vi "data_grid_v128_3d_plot.vi"(9 "No. Rows":i32=16, 10 "No. Columns":i32=8, 11 "Sensor Data":dbl[][](array[numeric])) -> (1 "Y (GRID)":dbl[][](array[numeric]), 2 "X (GRID)":dbl[][](array[numeric]), 3 "Z (GRID)":dbl[][](array[numeric]))   [LabVIEW 2018]
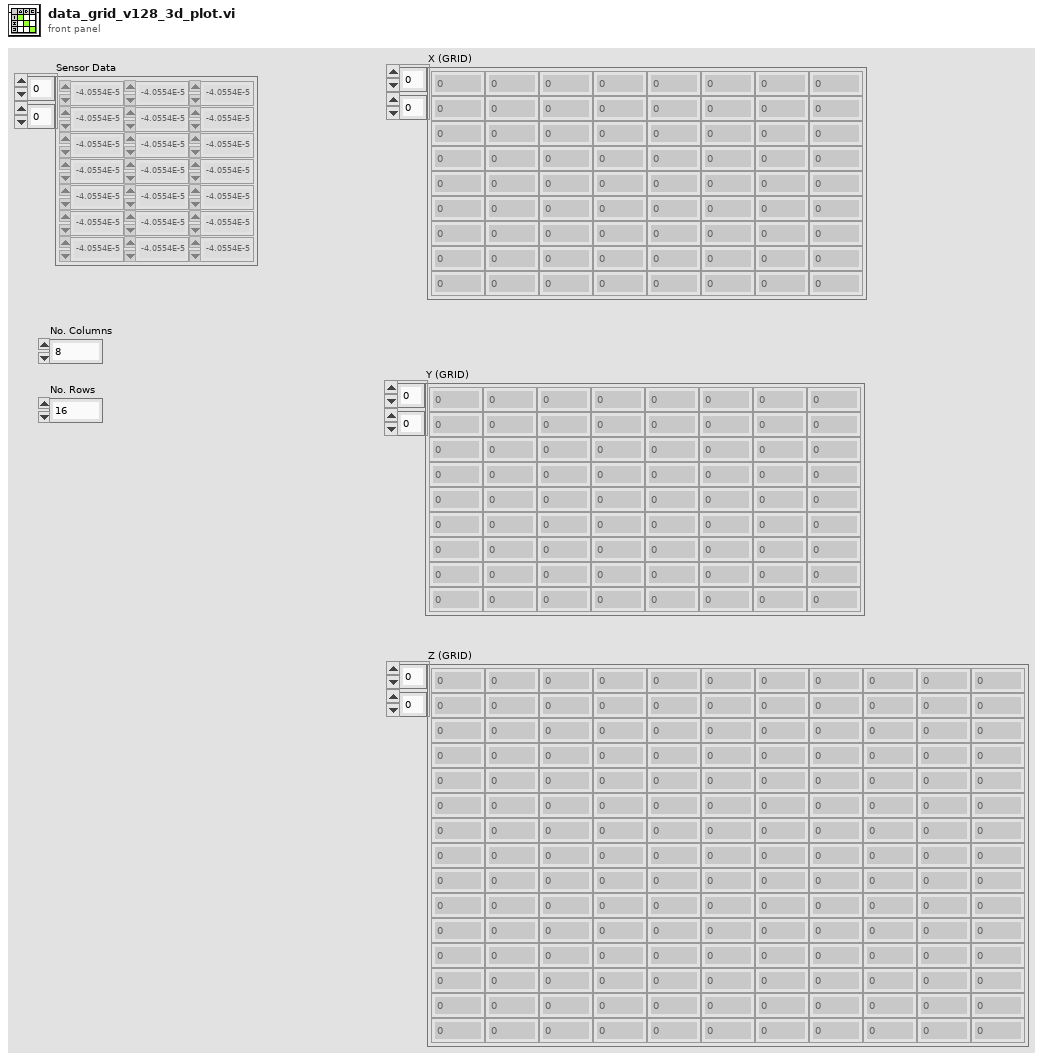
[diagram p1: front panel]
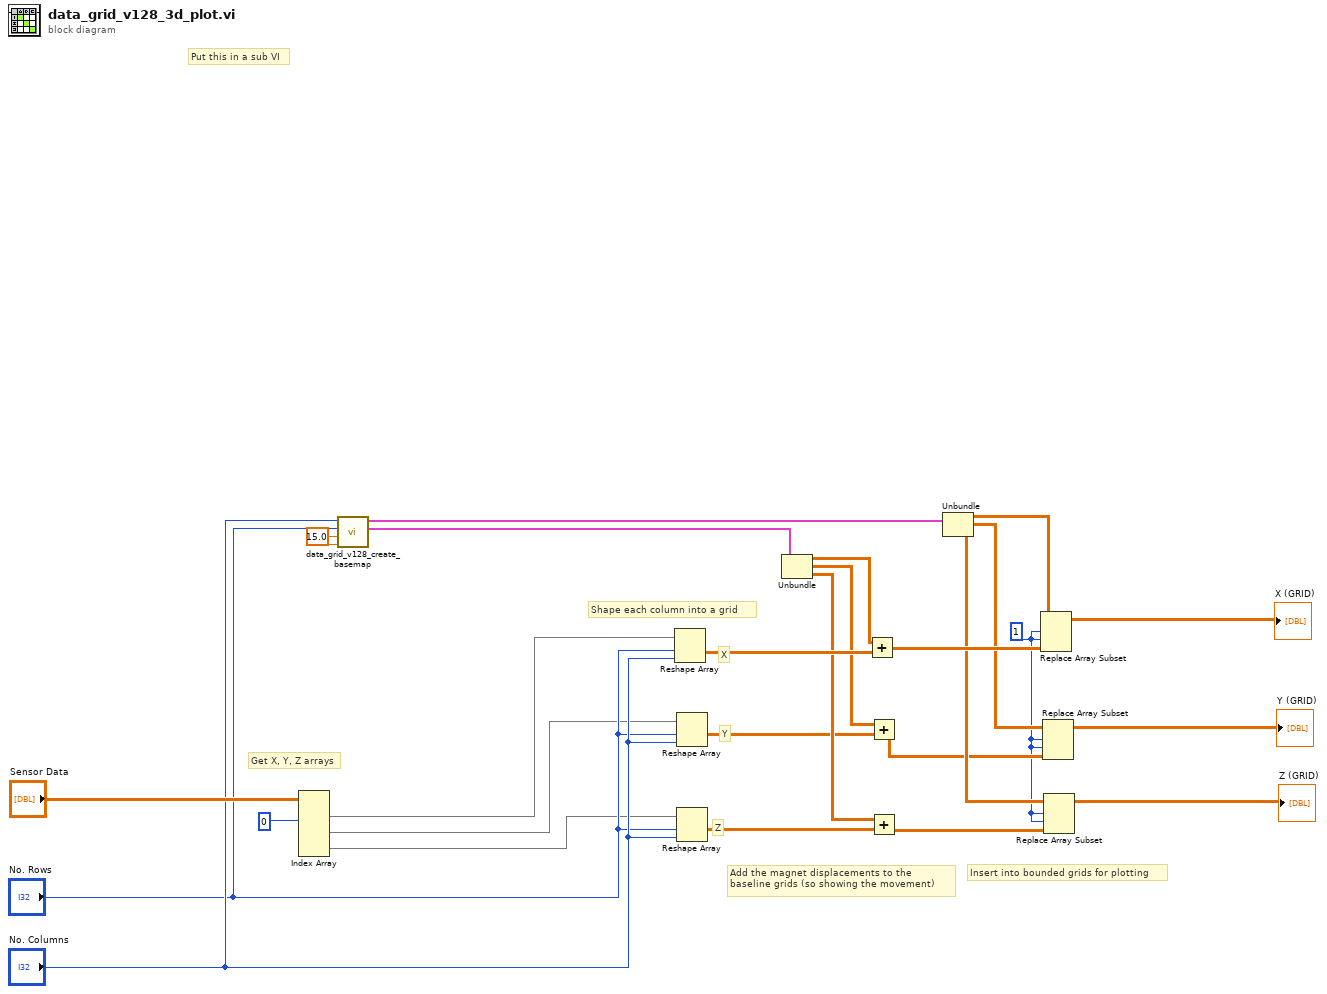
[diagram p0: block diagram]
diagram:
  w6 = 1 ("disabled index (col)")
  w21 = 15.0 ("X_spacing")
  # "Z"
  # "Y"
  # "X"
  # "Insert into bounded grids for plotting"
  # "Add the magnet displacements to the \nbaseline grids (so showing the movement)"
  # "Get X, Y, Z arrays"
  # "Shape each column into a grid"
  # "Put this in a sub VI"
  n1 = Index Array(array="Sensor Data", index (col) #1=0 ("disabled index (col)")) -> (element #1=w24:dbl[], element #2=w2:dbl[], element #3=w1:dbl[])  [unwired: 5 in]
  n2 = call "data_grid_v128_create_basemap.vi"("Y_spacing"=w21, "X_spacing"=w21, "No. Rows"="No. Rows", "No. Columns"="No. Columns") -> ("Grids_Unbounded"=w20:cluster{dbl[][], dbl[][], dbl[][]}, "Grids_Bounded"=w13:cluster{dbl[][], dbl[][], dbl[][]})  [unwired: 6 in]
  n3 = Reshape Array(w24, "No. Rows", "No. Columns") -> (w18:dbl[][])
  n4 = Reshape Array(w2, "No. Rows", "No. Columns") -> (w15:dbl[][])
  n5 = Reshape Array(w1, "No. Rows", "No. Columns") -> (w14:dbl[][])
  n6 = Unbundle(w20) -> (w19:dbl[][], w17:dbl[][], w16:dbl[][])
  n7 = Add(x=w19, y=w18) -> (x+y=w11:dbl[][])
  n8 = Add(x=w17, y=w15) -> (x+y=w8:dbl[][])
  n9 = Add(x=w16, y=w14) -> (x+y=w7:dbl[][])
  n10 = Unbundle(w13) -> (w12:dbl[][], w10:dbl[][], w9:dbl[][])
  n11 = Replace Array Subset(array=w12, new element=w11, index (row)=w6, index (col)=w6) -> (→"X (GRID)":dbl[][])
  n12 = Replace Array Subset(array=w10, new element=w8, index (row)=w6, index (col)=w6) -> (→"Y (GRID)":dbl[][])
  n13 = Replace Array Subset(array=w9, new element=w7, index (row)=w6, index (col)=w6) -> (→"Z (GRID)":dbl[][])
